vi "Chart[Template].Clear.vi"(8 "error in (no error)":errorcluster, 11 "DisplayWaveforms":refnum<class "DisplayWaveforms.lvclass">) -> (0 "error out":errorcluster, 3 "DisplayWaveforms out":refnum<class "DisplayWaveforms.lvclass">)   [LabVIEW 2020, in "DisplayWaveform.lvlib" / "DisplayWaveforms.lvclass"]
doc: "---------------------------------------------------------------\nJKI State Machine Objects™\nhttp://jki.net/state-machine-objects/\nCopyright (C) 2005-2015, JKI <info@jki.net>\nALL RIGHTS RESERVEDJKI State Machine Objects (SMO) 1.0.0.5\nJKI - JKI\nCopyright (c) 2016, JKI"
uses:
  DisplayWaveforms.lvclass
  DisplayWaveforms.lvclass/DisplayWaveforms.ctl
panel:
  # "For instructions on how to use the JKI State Machine Objects, examples and video tutorials, visit:\nhttp://jki.net/state-machine-objects/\n\nJKI State Machine Objects™\nhttp://jki.net/state-machine-objects/\nCopyright (C) 2005-2015, JKI <info@jki.net>\nALL RIGHTS RESERVED"
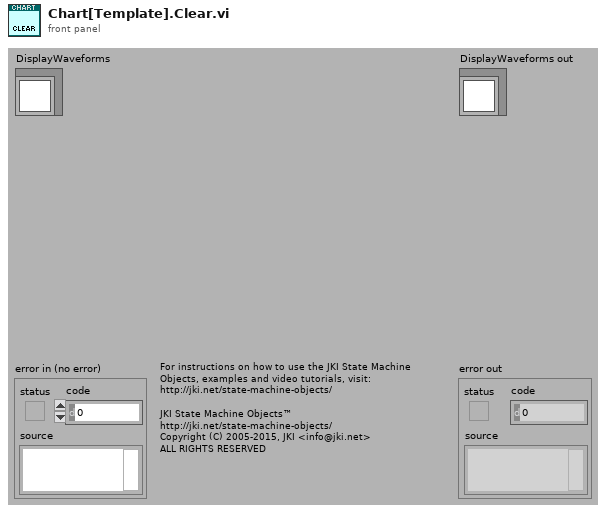
[diagram p1: front panel]
types:
  T1 = typedef "DisplayWaveform.lvlib/DisplayWaveforms.lvclass/PublicEvents--Cluster.ctl" = cluster{"Chart Cleared":refnum<user-event>, "Chart Paused":refnum<user-event>}
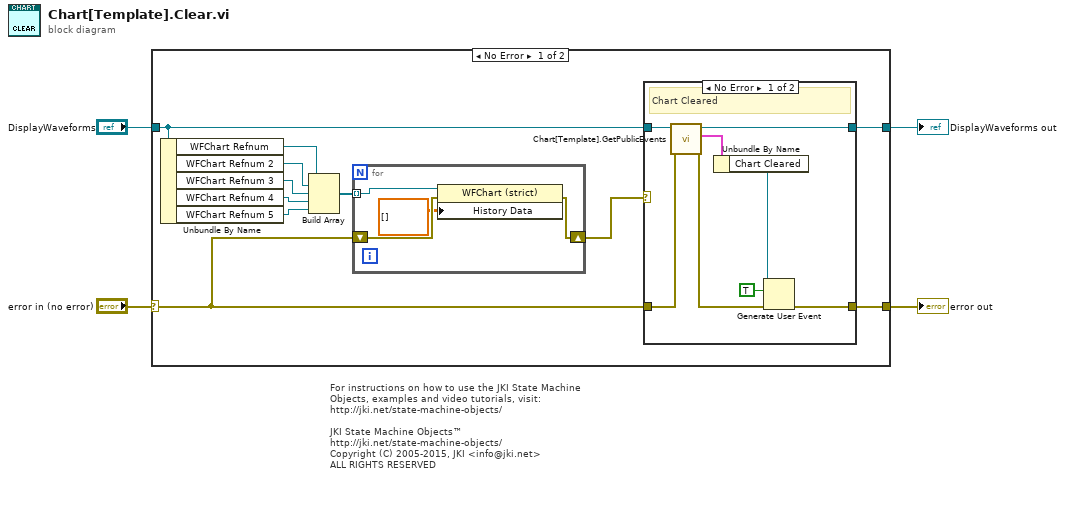
[diagram p0: block diagram]
diagram:
  # "For instructions on how to use the JKI State Machine Objects, examples and video tutorials, visit:\nhttp://jki.net/state-machine-objects/\n\nJKI State Machine Objects™\nhttp://jki.net/state-machine-objects/\nCopyright (C) 2005-2015, JKI <info@jki.net>\nALL RIGHTS RESERVED"
  n1 = case shown="No Error" "error in (no error)" {
    selector: "error in (no error)" -> [w5 w30]
    tunnel: "DisplayWaveforms" -> [w12 w31]
    tunnel: [w15 w30] -> w3
    tunnel: [w14 w31] -> w2
    frame No Error {
      n2 = Unbundle By Name(w12) -> ("WFChart Refnum"=w11:refnum<vi>, "WFChart Refnum 2"=w10:refnum<vi>, "WFChart Refnum 3"=w9:refnum<vi>, "WFChart Refnum 4"=w8:refnum<vi>, "WFChart Refnum 5"=w7:refnum<vi>)
      n3 = Build Array(w11, w10, w9, w8, w7) -> (w6:refnum<vi>[])
      n4 = for {
        tunnel: w6 -> [w18] mode=indexing
        shift-right: [w19] -> w13
        shift-left: w5 -> [w17]
        n5 = property class="WFChart (strict)"(reference=w18, error in=w17, "History Data"=dbl[][] []) -> (error out=w19:errorcluster)  [unwired: 1 out]
      }
      n6 = case shown="No Error" w13 {
        tunnel: w5 -> [w25 w28]
        tunnel: [w22 w28] -> w15
        tunnel: w12 -> [w27 w29]
        tunnel: [w26 w29] -> w14
        frame No Error {
          # "Chart Cleared"
          n7 = call "Chart[Template].GetPublicEvents.vi"("error in (no error)"=w25, "DisplayWaveforms"=w27) -> ("error out"=w23:errorcluster, "Chart[Template] Public Events"=w24:T1, "DisplayWaveforms out"=w26:refnum<class "DisplayWaveforms.lvclass">)  [unwired: 7 in]
          n8 = Unbundle By Name(w24) -> ("Chart Cleared"=w20:refnum<user-event>)
          n9 = Generate User Event(user event=w20, event data cluster=TRUE ("event data"), error in=w23) -> (error out=w22:errorcluster)  [unwired: 1 in, 1 out]
        }
        frame Error {
          # "Chart was not cleared"
        }
      }
    }
    frame Error {
    }
  }
  "error out" <- w3
  "DisplayWaveforms out" <- w2
